vi "Update Boolean.vi"(8 "error in (no error)":errorcluster, 10 "Boolean":bool, 11 "Business Logic in":refnum<class "Business Logic.lvclass">) -> (0 "error out":errorcluster, 3 "Business Logic out":refnum<class "Business Logic.lvclass">)   [LabVIEW 2020, in "Business Logic.lvlib" / "Business Logic.lvclass"]
uses:
  Business Logic.lvclass
  Business Logic.lvclass/Business Logic.ctl
  Indicators Messages/Update Boolean Msg/Update Boolean Msg.lvclass
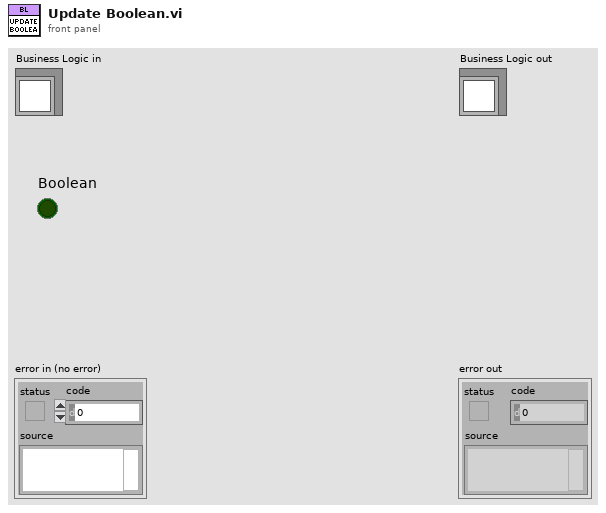
[diagram p1: front panel]
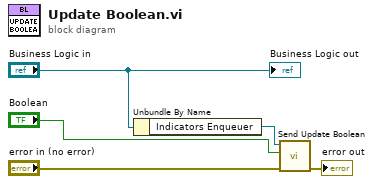
[diagram p0: block diagram]
diagram:
  n1 = Unbundle By Name("Business Logic in") -> ("Indicators Enqueuer"=w3:refnum<class "Message Enqueuer.lvclass">)
  n2 = call "Send Update Boolean.vi"("error in (no error)"="error in (no error)", "Boolean"="Boolean", "Message Enqueuer"=w3) -> ("error out"=→"error out":errorcluster)  [unwired: 7 in, 1 out]
  "Business Logic out" <- "Business Logic in"
